vi "Close Config Data.vi"(8 "error in (no error)":errorcluster, 10 "write file if changed (T)":bool=TRUE, 11 "refnum":T1) -> (0 "error out":errorcluster, 3 "file path":path)   [LabVIEW 2017, in "NI_LVConfig.lvlib"]
doc: "Writes data to the platform-independent configuration file identified by <B>refnum</B> and then closes the reference to that file."
uses:
  <vilib>/Utility/config.llb/NI_LVConfig.lvlib
  <vilib>/Utility/config.llb/Config Data RefNum.ctl
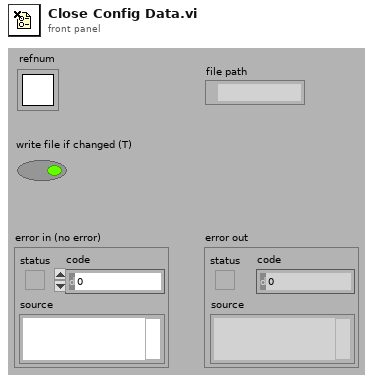
[diagram p1: front panel]
types:
  T1 = typedef "NI_LVConfig.lvlib/Config Data RefNum.ctl" = refnum<k1>
  T2 = typedef "NI_LVConfig.lvlib/Config Queue.ctl" = refnum<queue>
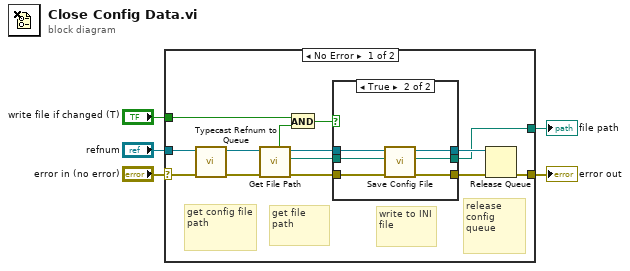
[diagram p0: block diagram]
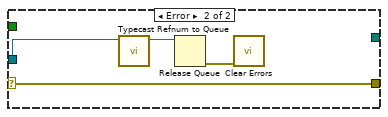
[diagram p3: hidden frame]
diagram:
  n1 = case shown="No Error" "error in (no error)" {
    selector: "error in (no error)" -> [w15 w31]
    tunnel: "refnum" -> [w11 w30]
    tunnel: "write file if changed (T)" -> [w17 _]
    tunnel: [w12 w31] -> w3
    tunnel: [w6 _] -> w2
    frame No Error {
      # "release config queue"
      # "write to INI file"
      # "get file path"
      # "get config file path"
      n2 = call <vilib>:"Typecast Refnum to Queue.vi"("refnum in"=w11) -> ("queue out"=w10:T2)  [unwired: 10 in]
      n3 = call <vilib>:"Get File Path.vi"("error in (no error)"=w15, "queue in"=w10) -> ("error out"=w8:errorcluster, "file path"=w7:path, "queue out"=w16:T2, "need update"=w9:bool)  [unwired: 1 in, 5 out]
      n4 = And(x=w17, y=w9) -> (x .and. y?=w18:bool)
      n5 = case shown="True" w18 {
        tunnel: w8 -> [w21 w26]
        tunnel: w16 -> [w20 w27]
        tunnel: [w21 w25] -> w13
        tunnel: [w20 w24] -> w14
        tunnel: w7 -> [w19 w23]
        tunnel: [w19 w22] -> w6
        frame False {
        }
        frame True {
          n6 = call <vilib>:"Save Config File.vi"("error in (no error)"=w26, "file path"=w23, "queue in"=w27) -> ("error out"=w25:errorcluster, "file path out"=w22:path, "queue out"=w24:T2)  [unwired: 6 out]
        }
      }
      n7 = Release Queue(queue=w14, error in (no error)=w13) -> (error out=w12:errorcluster)  [unwired: 1 in, 2 out]
    }
    frame Error {
      n8 = call <vilib>:"Typecast Refnum to Queue.vi"("refnum in"=w30) -> ("queue out"=w29:T2)  [unwired: 10 in]
      n9 = Release Queue(queue=w29) -> (error out=w28:errorcluster)  [unwired: 2 in, 2 out]
      n10 = call <vilib>:"Clear Errors.vi"("error in (no error)"=w28) -> ()  [unwired: 5 in, 2 out]
    }
  }
  "error out" <- w3
  "file path" <- w2
